vi "Actor Core.vi"(8 "error in":errorcluster, 11 "Nested in":refnum<class "UI.lvclass">) -> (0 "error out":errorcluster, 3 "Actor out":refnum<class "Actor.lvclass">)   [LabVIEW 2020, in "UI.lvlib" / "UI.lvclass"]
doc: "(<B>Filename</B>: Actor Framework.lvlib:Actor.lvclass:Actor Core.vi)\n\nReceives messages to the actor, reacts to them, and initiates any error handling that may shut the actor down.\n\nDescendant classes may override this VI to append parallel tasks for the actor to complete while it handles messages. Overrides use the Call Parent Method node."
uses:
  UI.lvclass
  C:/Program Files (x86)/National Instruments/LabVIEW 2020/vi.lib/ActorFramework/Actor/Actor.lvclass
  <vilib>/ActorFramework/Actor/Actor.lvclass
  <vilib>/ActorFramework/Actor/Actor.lvclass/Actor.ctl
  <vilib>/ActorFramework/Message Enqueuer/Message Enqueuer.lvclass/Message Enqueuer.ctl
  UI.lvclass/UI.ctl
  Read Serial Device.lvclass.vi
  Read VISA resource name.vi
  <vilib>/ActorFramework/Message Enqueuer/Init from Existing Queue.vi
  <vilib>/ActorFramework/Message Enqueuer/Enqueue.vi
  <vilib>/ActorFramework/Stop Msg/Stop Msg.lvclass
  C:/Program Files (x86)/National Instruments/LabVIEW 2020/vi.lib/ActorFramework/Message/Message.lvclass
  <vilib>/ActorFramework/Message Priority Queue/Priority Enqueue.vi
  <vilib>/ActorFramework/Message Enqueuer/Message Enqueuer.lvclass
  Abstract/Serial Device/Serial Device.lvclass
panel:
  out "VISA resource name":refnum<visa-resource-name>
  in  "Read ADC":bool
  in  "Channel ADC":u16
  out "Value":dbl(slide) scale=0.0..10.0
  in  "Port":u16
  in  "Set Port":bool[](array[boolean])
  in  "Set Port Status":bool
  in  "Port 2":dbl
  out "Get Port":bool[](array[boolean])
  in  "Get Port Status":bool
  in  "Port 3":dbl
  in  "Set Pin":bool
  in  "Pin":dbl
  in  "Set Pin Status":bool
  in  "Port 4":dbl
  out "Get Pin":bool
  in  "Pin 2":dbl
  in  "Get Pin Status":bool
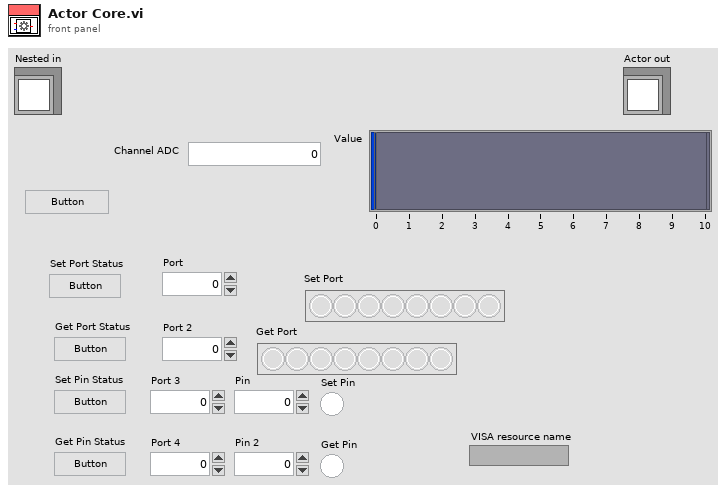
[diagram p1: front panel]
types:
  T1 = cluster{"Stop":refnum<user-event>, "Value ":refnum<user-event>, "Set Port":refnum<user-event>, "Get Port":refnum<user-event>, "Get Pin":refnum<user-event>}
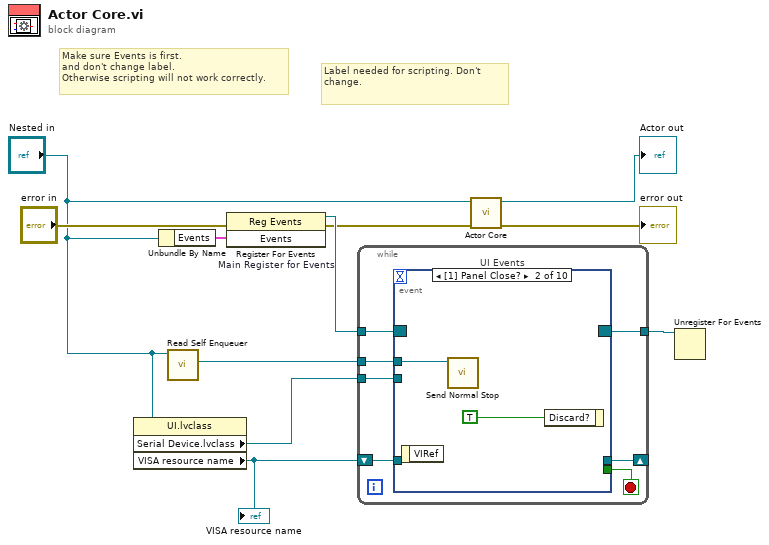
[diagram p0: block diagram]
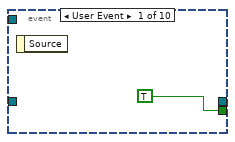
[diagram p2: hidden frame]
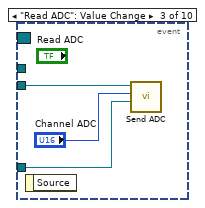
[diagram p3: hidden frame]
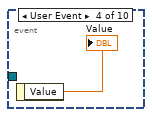
[diagram p4: hidden frame]
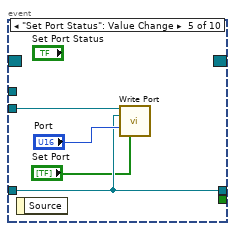
[diagram p5: hidden frame]
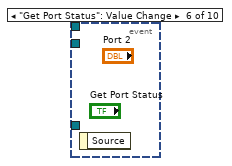
[diagram p6: hidden frame]
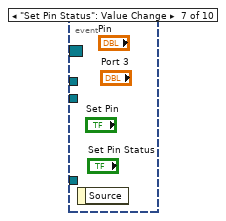
[diagram p7: hidden frame]
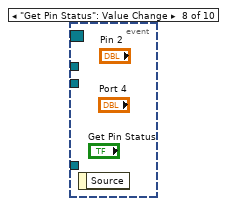
[diagram p8: hidden frame]
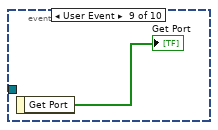
[diagram p9: hidden frame]
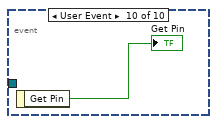
[diagram p10: hidden frame]
diagram:
  # "Label needed for scripting. Don't change."
  # "Make sure Events is first.\nand don't change label.\nOtherwise scripting will not work correctly."
  n1 = property class="UI.lvclass"(reference="Nested in") -> ("Serial Device.lvclass"=w2:refnum<class "Serial Device.lvclass">, "VISA resource name"=w1:refnum<visa-resource-name>)  [unwired: 1 in, 2 out]
  "VISA resource name" <- w1
  n2 = Unbundle By Name("Nested in") -> ("Events"=w8:T1)
  n3 = call <vilib>:"Read Self Enqueuer.vi"("Actor"="Nested in") -> ("Self Enqueuer"=w6:refnum<class "Message Enqueuer.lvclass">)  [unwired: 10 in]
  n4 = register-events "Main Register for Events"(error in="error in", w8) -> (reference out=w9:refnum<event-registration>, error out=w4:errorcluster)  [unwired: 1 in]
  n5 = while {
    tunnel: w9 -> [w18]
    tunnel: [w16] -> w7
    tunnel: w6 -> [w15]
    tunnel: w2 -> [w14]
    shift-right: [w12] -> _
    shift-left: w1 -> [w13]
    stop <- w17 stop-if-true
    n6 = event "UI Events" shown="[1] Panel Close?" {
      selector: w18 -> [_ _ _ _ _ _ _ _ _ _]
      dyn-events: [_ _ _ _ _ _ _ _ _ _] -> w16
      timeout: _ -> [_ _ _ _ _ _ _ _ _ _]
      tunnel: [TRUE _ _ _ _ _ _ _ _ _] -> w17
      tunnel: w15 -> [_ w20 _ _ _ _ _ _ _ _]
      tunnel: w14 -> [_ _ w24 _ w29 _ _ _ _ _]
      tunnel: w13 -> [_ _ w22 _ w27 _ _ _ _ _]
      tunnel: [_ _ _ _ w27 _ _ _ _ _] -> w12
      event User Event {
        n7 = event-data() -> ()  [unwired: 1 in, 1 out]
      }
      event Panel Close? {
        n8 = event-data() -> ()  [unwired: 1 in, 1 out]
        n9 = call <vilib>:"Send Normal Stop.vi"("Message Enqueuer"=w20) -> ()  [unwired: 10 in, 1 out]
        n10 = event-data("Discard?"=TRUE) -> ()  [unwired: 1 in, 1 out]
      }
      event "Read ADC": Value Change {
        n11 = event-data() -> ()  [unwired: 1 in, 1 out]
        n12 = call-dynamic "Send ADC.vi"("VISA resource name"=w22, "Channel ADC"="Channel ADC", "Serial Device in"=w24) -> ()  [unwired: 7 in, 2 out]
      }
      event User Event {
        n13 = event-data() -> ("Value"=→"Value":dbl)  [unwired: 1 in]
      }
      event "Set Port Status": Value Change {
        n14 = event-data() -> ()  [unwired: 1 in, 1 out]
        n15 = call-dynamic "Write Port.vi"("Serial Device in"=w29, "VISA resource name"=w27, "Port"="Port", "Set Port"="Set Port") -> ()  [unwired: 9 in, 3 out]
      }
      event "Get Port Status": Value Change {
        n16 = event-data() -> ()  [unwired: 1 in, 1 out]
      }
      event "Set Pin Status": Value Change {
        n17 = event-data() -> ()  [unwired: 1 in, 1 out]
      }
      event "Get Pin Status": Value Change {
        n18 = event-data() -> ()  [unwired: 1 in, 1 out]
      }
      event User Event {
        n19 = event-data() -> ("Get Port"=→"Get Port":bool[])  [unwired: 1 in]
      }
      event User Event {
        n20 = event-data() -> ("Get Pin"=→"Get Pin":bool)  [unwired: 1 in]
      }
    }
  }
  n21 = call-parent "Actor Core.vi"("error in"=w4, "Actor in"="Nested in") -> ("error out"=→"error out":errorcluster, "Actor out"=→"Actor out":refnum<class "Actor.lvclass">)  [unwired: 8 in]
  n22 = Unregister For Events(event registration refnum=w7) -> ()  [unwired: 1 in, 1 out]
